vi "Get Steering Frame Velocity from Wheels.vi"(5 "wheel indexes":i32[](array[numeric]), 7 "get motor data (F)":bool, 8 "error in (no error)":errorcluster, 9 "acquired wheel states":T1[](array[typedef]), 11 "steering frame in":refnum<class "NI_Robotics_Steering Frame.lvclass">) -> (0 "error out":errorcluster, 1 "wheel states":T1[](array[typedef]), 2 "estimated steering frame velocity":dbl[](array[numeric]), 3 "steering frame out":refnum<class "NI_Robotics_Steering Frame.lvclass">)   [LabVIEW 2017, in "NI_Robotics_Steering Frame.lvclass"]
doc: "Calculates the steering frame velocity or arc velocity required to best satisfy the state of each wheel. You can read data for each wheel from wheel motors or specify the wheel data manually. You must manually select the polymorphic instance to use."
uses:
  <vilib>/robotics/Steering/Steering Frame/NI_Robotics_Steering Frame.lvclass
  <vilib>/robotics/Steering/Wheel/Wheel State.ctl
  <vilib>/robotics/Steering/Steering Frame/NI_Robotics_Steering Frame.lvclass/NI_Robotics_Steering Frame.ctl
  <vilib>/robotics/Utilities/Generate Error.vi
  <vilib>/robotics/Steering/Steering Frame/Merge Wheel States.vi
  <vilib>/robotics/Steering/Wheel/Read Wheel State from Motors.vi
  <vilib>/robotics/Steering/Wheel/Create Wheel Angular Velocity Row_Frame.vi
  <vilib>/robotics/Steering/Wheel/Create Caster Angular Velocity Row_Frame.vi
  <vilib>/robotics/Steering/Wheel/Set Current Caster Angle_Frame.vi
  <vilib>/Analysis/7linalg.llb/Solve General Linear Equations with SVD (DBL).vi
  <vilib>/robotics/Steering/Wheel/NI_Robotics_Wheel.lvclass
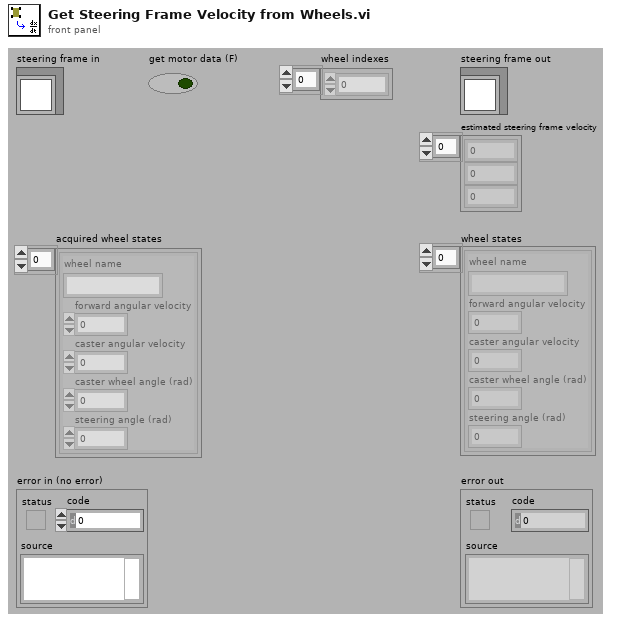
[diagram p1: front panel]
types:
  T1 = typedef "NI_Robotics_Wheel.lvclass/Wheel State.ctl" = cluster{"wheel name":string, "forward angular velocity":dbl, "caster angular velocity":dbl, "caster wheel angle (rad)":dbl, "steering angle (rad)":dbl}
  T2 = cluster{"wheel index (all)":i32, "wheel index (used)":i32, "wheels used":i32}
  T3 = typedef "NI_Matrix.lvlib/RealMatrix.ctl" = dbl[][]
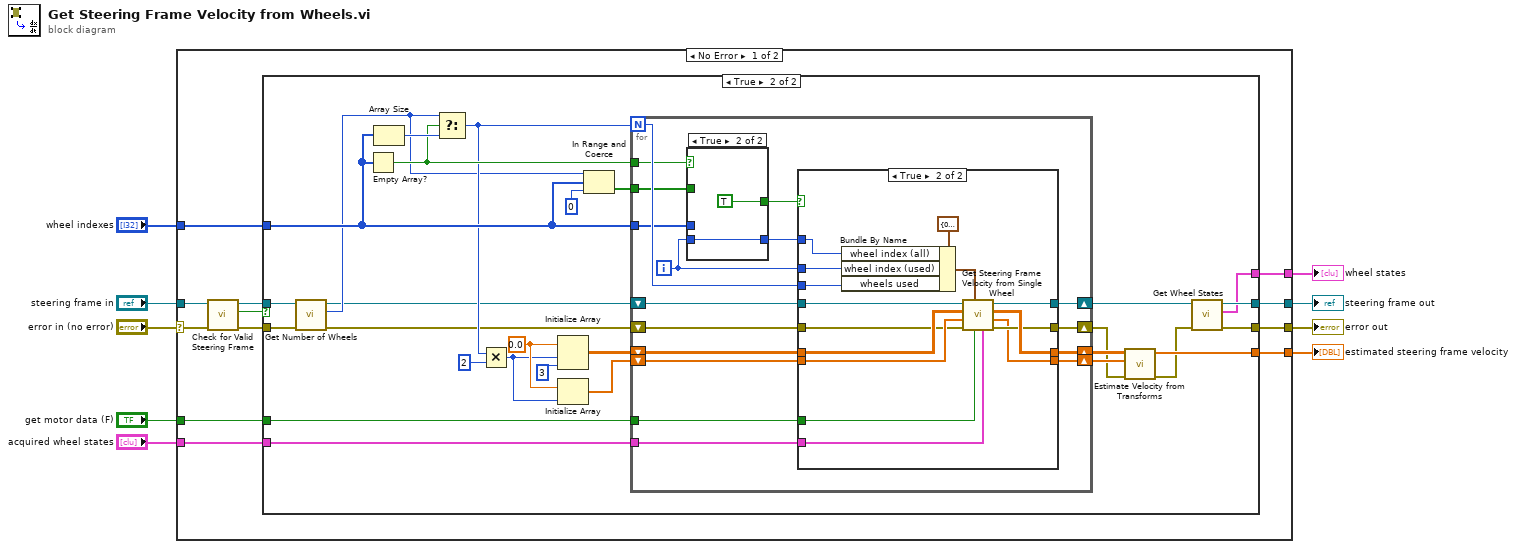
[diagram p0: block diagram]
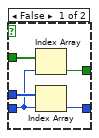
[diagram p4: hidden frame]
diagram:
  n1 = case shown="No Error" "error in (no error)" {
    selector: "error in (no error)" -> [w14 w96]
    tunnel: [w20 w96] -> w8
    tunnel: [w18 w95] -> w6
    tunnel: "steering frame in" -> [w16 w95]
    tunnel: [w21 _] -> w5
    tunnel: "acquired wheel states" -> [w19 _]
    tunnel: "get motor data (F)" -> [w17 _]
    tunnel: [w11 _] -> w2
    tunnel: "wheel indexes" -> [w10 _]
    frame No Error {
      n2 = call <vilib>:"Check for Valid Steering Frame.vi"("error in (no error)"=w14, "steering frame in"=w16) -> ("error out"=w13:errorcluster, "valid?"=w12:bool, "steering frame out"=w15:refnum<class "NI_Robotics_Steering Frame.lvclass">)  [unwired: 7 in]
      n3 = case shown="True" w12 {
        tunnel: [_ w27] -> w21
        tunnel: [w22 w24] -> w20
        tunnel: w19 -> [_ w50]
        tunnel: [w23 w48] -> w18
        tunnel: w17 -> [_ w51]
        tunnel: w15 -> [w23 w33]
        tunnel: w13 -> [w22 w31]
        tunnel: [_ w47] -> w11
        tunnel: w10 -> [_ w49]
        frame False {
        }
        frame True {
          w37 = 0.0 ("element")
          n4 = call <vilib>:"Get Number of Wheels.vi"("error in (no error)"=w31, "steering frame in"=w33) -> ("error out"=w30:errorcluster, "number of wheels"=w34:i32, "steering frame out"=w32:refnum<class "NI_Robotics_Steering Frame.lvclass">)  [unwired: 7 in]
          n5 = Empty Array?(array=w49) -> (empty?=w42:bool)
          n6 = Array Size(array=w49) -> (size(s)=w45:i32)
          n7 = Select(t=w34, s=w42, f=w45) -> (s? t:f=w41:i32)
          n8 = Multiply(x=w41, y=2) -> (x*y=w36:i32)
          n9 = Initialize Array(w37, w36, 3 ("dimension size")) -> (w38:dbl[][])
          n10 = Initialize Array(w37, w36) -> (w35:dbl[])
          n11 = In Range and Coerce(upper limit=w34, x=w49, lower limit=0) -> (In Range?=w43:bool[])  [unwired: 1 out]
          n12 = for {
            N: w41 -> [w60]
            shift-right: [w62] -> w29
            shift-left: w38 -> [w63]
            shift-right: [w68] -> w26
            shift-left: w30 -> [w67]
            tunnel: w51 -> [w66]
            shift-right: [w64] -> w28
            shift-left: w35 -> [w65]
            tunnel: w50 -> [w61]
            tunnel: w49 -> [w59]
            tunnel: w43 -> [w58]
            tunnel: w42 -> [w55]
            shift-right: [w53] -> w46
            shift-left: w32 -> [w54]
            i -> [w52]
            n13 = case shown="True" w55 {
              tunnel: w59 -> [w92 _]
              tunnel: w52 -> [w90 w94]
              tunnel: [w89 w94] -> w57
              tunnel: w58 -> [w91 _]
              tunnel: [w88 TRUE ("lower limit")] -> w56
              frame False {
                n14 = Index Array(array=w91, index=w90) -> (element=w88:bool)
                n15 = Index Array(array=w92, index=w90) -> (element=w89:i32)
              }
              frame True {
              }
            }
            n16 = case shown="True" w56 {
              tunnel: [w69 w82] -> w68
              tunnel: w67 -> [w69 w83]
              tunnel: w66 -> [_ w81]
              tunnel: w65 -> [w70 w84]
              tunnel: [w70 w79] -> w64
              tunnel: w63 -> [w72 w86]
              tunnel: [w72 w85] -> w62
              tunnel: w61 -> [_ w80]
              tunnel: w60 -> [_ w73]
              tunnel: w57 -> [_ w75]
              tunnel: w54 -> [w71 w87]
              tunnel: [w71 w78] -> w53
              tunnel: w52 -> [_ w74]
              frame False {
              }
              frame True {
                n17 = Bundle By Name(cluster=T2 {"wheel index (all)"=0, "wheel index (used)"=0, "wheels used"=0} ("index info"), "wheel index (all)"=w75, "wheel index (used)"=w74, "wheels used"=w73) -> (w76:T2)
                n18 = call <vilib>:"Get Steering Frame Velocity from Single Wheel.vi"("acquired wheel states"=w80, "get motor data"=w81, "index info"=w76, "error in (no error)"=w83, "velocity transform vector in"=w84, "velocity transform matrix in"=w86, "steering frame in"=w87) -> ("error out"=w82:errorcluster, "velocity transform vector out"=w79:dbl[], "velocity transform matrix out"=w85:T3, "steering frame out"=w78:refnum<class "NI_Robotics_Steering Frame.lvclass">)  [unwired: 1 in]
              }
            }
          }
          n19 = call <vilib>:"Estimate Velocity from Transforms.vi"("error in (no error)"=w26, "velocity transform vector in"=w28, "velocity transform matrix in"=w29) -> ("error out"=w25:errorcluster, "estimated steering frame velocity"=w27:dbl[])  [unwired: 7 in]
          n20 = call <vilib>:"Get Wheel States.vi"("error in (no error)"=w25, "steering frame in"=w46) -> ("error out"=w24:errorcluster, "wheel states"=w47:T1[], "steering frame out"=w48:refnum<class "NI_Robotics_Steering Frame.lvclass">)  [unwired: 7 in]
        }
      }
    }
    frame Error {
    }
  }
  "error out" <- w8
  "steering frame out" <- w6
  "estimated steering frame velocity" <- w5
  "wheel states" <- w2
